vi "DESTUE.vi"(8 "error in (no error)":errorcluster, 11 "CONTADOR_CON_LIMITES in":refnum<class "CONTADOR_CON_LIMITES.lvclass">) -> (0 "error out":errorcluster, 3 "CONTADOR_CON_LIMITES out":refnum<class "CONTADOR_CON_LIMITES.lvclass">)   [LabVIEW 2019, in "CONTADOR_CON_LIMITES.lvlib" / "CONTADOR_CON_LIMITES.lvclass"]
uses:
  CONTADOR_CON_LIMITES.lvclass
  CONTADOR_CON_LIMITES.lvclass/CONTADOR_CON_LIMITES.ctl
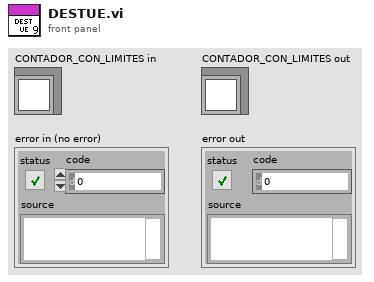
[diagram p1: front panel]
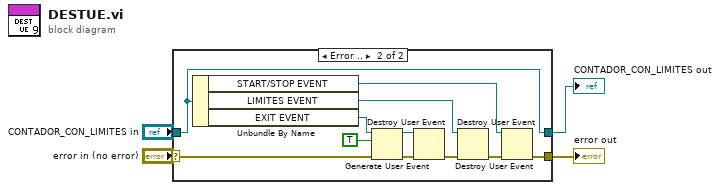
[diagram p0: block diagram]
diagram:
  n1 = case shown="Error .." "error in (no error)" {
    selector: "error in (no error)" -> [w5 w15]
    tunnel: "CONTADOR_CON_LIMITES in" -> [w6 w7]
    tunnel: [w6 w7] -> w3
    tunnel: [w5 w8] -> w4
    frame No Error {
    }
    frame Error {
      n2 = Unbundle By Name(w7) -> ("START/STOP EVENT"=w11:refnum<user-event>, "LIMITES EVENT"=w12:refnum<user-event>, "EXIT EVENT"=w17:refnum<user-event>)
      n3 = Generate User Event(user event=w17, event data cluster=TRUE ("event data"), error in=w15) -> (user event out=w13:refnum<user-event>, error out=w14:errorcluster)  [unwired: 1 in]
      n4 = Destroy User Event(user event=w13, error in=w14) -> (error out=w10:errorcluster)
      n5 = Destroy User Event(user event=w12, error in=w10) -> (error out=w9:errorcluster)
      n6 = Destroy User Event(user event=w11, error in=w9) -> (error out=w8:errorcluster)
    }
  }
  "error out" <- w4
  "CONTADOR_CON_LIMITES out" <- w3
